vi "Userinterface_BP_MC1.vi"() -> ()   [LabVIEW 2010]
uses:
  <vilib>/addons/Simulation Interface/_sitctls/sit Indicator Info.ctl
  <vilib>/addons/Simulation Interface/_sitctls/sit Indicator Type.ctl
  <vilib>/addons/Simulation Interface/_sitctls/sit Client Meta Info (v3).ctl
  <vilib>/addons/Simulation Interface/_sitctls/sit MDL Line Item Info.ctl
  <vilib>/addons/Simulation Interface/_sitctls/sit MDL Line Type.ctl
  <vilib>/addons/Simulation Interface/_sitctls/sit Details Settings.ctl
  <vilib>/addons/Simulation Interface/_sitctls/sit Execution Host.ctl
  <vilib>/addons/Simulation Interface/_sitctls/SIT Sim State.ctl
  <vilib>/Utility/inputDevices.llb/closeJoystick.vi
  <vilib>/Utility/inputDevices.llb/joystickAcquire.vi
  <vilib>/addons/Simulation Interface/_sitclient.llb/NI_SIT_sitclient.lvlib
  <vilib>/addons/Simulation Interface/_sitctls/NI_SIT_sitctls.lvlib
  <vilib>/ptbypt/NI_PtbyPt.lvlib
panel:
  out "Left Joystick":bool
  out "Right Joystick":bool
  in  "R2":sgl
  in  "L2":sgl
  out "Direction Up":bool
  out "Direction Right":bool
  out "Direction Down":bool
  out "Direction Left":bool
  out "L2 Button":bool
  out "R2 Button":bool
  out "Triangle Button":bool
  out "Circle Button":bool
  out "X Button":bool
  out "Square Button":bool
  out "Joystick Info":T1(array[cluster])
  in  "VSP Speed":dbl(slide) min=-1.0 max=1.0 step=0.05 scale=-1.0..1.0 scale format="%#_2g"
  in  "Power Limiter":dbl(slide) min=0.0 max=1.0 step=0.1 scale=-1.0..1.0
  in  "Left Y":dbl(slide) scale=-35860.0..35860.0
  in  "Left X":dbl(slide) scale=-35860.0..35860.0
  in  "Right X":dbl(slide) scale=-35860.0..35860.0
  in  "Right Y":dbl(slide) scale=-35860.0..35860.0
  in  "SIT_Meta_Info":T2={"Simulation IP"="localhost", "Target IP"="192.168.0.77", "Host Port"=6011, "Model DLL Path"=path "C:/Documents and Settings/mcl/Desktop/CSE Manual Controll/BP_MC1_nidll_rtw/BP_MC1.dll", "Model File Path"=path "C:/Documents and Settings/mcl/Desktop/CSE Manual Controll/BP_MC1_nidll_rtw/BP_MC1.dll", "Model Name"="bp_mc1", "Param Tree Info "=[{"Line Type"=enum."Section Head", "Section Type"="Model", "Name"="bp_mc1", "Value"="", "Owner Index"=-3, "Tree Tag"="", "Child Indices"=[1, 6, 27], "Expanded?"=FALSE, "Destination Block Info"=[]}, {"Line Type"=enum."Section Head", "Section Type"="Subsystem", "Name"="Labview Output", "Value"="", "Owner Index"=0, "Tree Tag"="", "Child Indices"=[2, 4], "Expanded?"=FALSE, "Destination Block Info"=[]}, {"Line Type"=enum."Section Head", "Section Type"="Subsystem", "Name"="LabVIEW_BT_Limit", "Value"="", "Owner Index"=1, "Tree Tag"="", "Child Indices"=[3], "Expanded?"=FALSE, "Destination Block Info"=[]}, {"Line Type"=enum."Parameter", "Section Type"="", "Name"="Value", "Value"="", "Owner Index"=2, "Tree Tag"="", "Child Indices"=[], "Expanded?"=FALSE, "Destination Block Info"=[]}, {"Line Type"=enum."Section Head", "Section Type"="Subsystem", "Name"="LabVIEW_VSPS", "Value"="", "Owner Index"=1, "Tree Tag"="", "Child Indices"=[5], "Expanded?"=FALSE, "Destination Block Info"=[]}, {"Line Type"=enum."Parameter", "Section Type"="", "Name"="Value", "Value"="", "Owner Index"=4, "Tree Tag"="", "Child Indices"=[], "Expanded?"=FALSE, "Destination Block Info"=[]}, {"Line Type"=enum."Section Head", "Section Type"="Subsystem", "Name"="PS3 Controller Output", "Value"="", "Owner Index"=0, "Tree Tag"="", "Child Indices"=[7, 9, 11, 13, 15, 17, 19, 21, 23, 25], "Expanded?"=FALSE, "Destination Block Info"=[]}, {"Line Type"=enum."Section Head", "Section Type"="Subsystem", "Name"="JS_L_X", "Value"="", "Owner Index"=6, "Tree Tag"="", "Child Indices"=[8], "Expanded?"=FALSE, "Destination Block Info"=[]}, {"Line Type"=enum."Parameter", "Section Type"="", "Name"="Value", "Value"="", "Owner Index"=7, "Tree Tag"="", "Child Indices"=[], "Expanded?"=FALSE, "Destination Block Info"=[]}, {"Line Type"=enum."Section Head", "Section Type"="Subsystem", "Name"="JS_L_Y", "Value"="", "Owner Index"=6, "Tree Tag"="", "Child Indices"=[10], "Expanded?"=FALSE, "Destination Block Info"=[]}, {"Line Type"=enum."Parameter", "Section Type"="", "Name"="Value", "Value"="", "Owner Index"=9, "Tree Tag"="", "Child Indices"=[], "Expanded?"=FALSE, "Destination Block Info"=[]}, {"Line Type"=enum."Section Head", "Section Type"="Subsystem", "Name"="JS_R_X", "Value"="", "Owner Index"=6, "Tree Tag"="", "Child Indices"=[12], "Expanded?"=FALSE, "Destination Block Info"=[]}, {"Line Type"=enum."Parameter", "Section Type"="", "Name"="Value", "Value"="", "Owner Index"=11, "Tree Tag"="", "Child Indices"=[], "Expanded?"=FALSE, "Destination Block Info"=[]}, {"Line Type"=enum."Section Head", "Section Type"="Subsystem", "Name"="JS_R_Y", "Value"="", "Owner Index"=6, "Tree Tag"="", "Child Indices"=[14], "Expanded?"=FALSE, "Destination Block Info"=[]}, {"Line Type"=enum."Parameter", "Section Type"="", "Name"="Value", "Value"="", "Owner Index"=13, "Tree Tag"="", "Child Indices"=[], "Expanded?"=FALSE, "Destination Block Info"=[]}, {"Line Type"=enum."Section Head", "Section Type"="Subsystem", "Name"="L2", "Value"="", "Owner Index"=6, "Tree Tag"="", "Child Indices"=[16], "Expanded?"=FALSE, "Destination Block Info"=[]}, {"Line Type"=enum."Parameter", "Section Type"="", "Name"="Value", "Value"="", "Owner Index"=15, "Tree Tag"="", "Child Indices"=[], "Expanded?"=FALSE, "Destination Block Info"=[]}, {"Line Type"=enum."Section Head", "Section Type"="Subsystem", "Name"="R2", "Value"="", "Owner Index"=6, "Tree Tag"="", "Child Indices"=[18], "Expanded?"=FALSE, "Destination Block Info"=[]}, {"Line Type"=enum."Parameter", "Section Type"="", "Name"="Value", "Value"="", "Owner Index"=17, "Tree Tag"="", "Child Indices"=[], "Expanded?"=FALSE, "Destination Block Info"=[]}, {"Line Type"=enum."Section Head", "Section Type"="Subsystem", "Name"="Scaling_JS_L_X", "Value"="", "Owner Index"=6, "Tree Tag"="", "Child Indices"=[20], "Expanded?"=FALSE, "Destination Block Info"=[]}, {"Line Type"=enum."Parameter", "Section Type"="", "Name"="Gain", "Value"="", "Owner Index"=19, "Tree Tag"="", "Child Indices"=[], "Expanded?"=FALSE, "Destination Block Info"=[]}, {"Line Type"=enum."Section Head", "Section Type"="Subsystem", "Name"="Scaling_JS_L_Y", "Value"="", "Owner Index"=6, "Tree Tag"="", "Child Indices"=[22], "Expanded?"=FALSE, "Destination Block Info"=[]}, {"Line Type"=enum."Parameter", "Section Type"="", "Name"="Gain", "Value"="", "Owner Index"=21, "Tree Tag"="", "Child Indices"=[], "Expanded?"=FALSE, "Destination Block Info"=[]}, {"Line Type"=enum."Section Head", "Section Type"="Subsystem", "Name"="Scaling_JS_R_X", "Value"="", "Owner Index"=6, "Tree Tag"="", "Child Indices"=[24], "Expanded?"=FALSE, "Destination Block Info"=[]}, {"Line Type"=enum."Parameter", "Section Type"="", "Name"="Gain", "Value"="", "Owner Index"=23, "Tree Tag"="", "Child Indices"=[], "Expanded?"=FALSE, "Destination Block Info"=[]}, {"Line Type"=enum."Section Head", "Section Type"="Subsystem", "Name"="Scaling_JS_R_Y", "Value"="", "Owner Index"=6, "Tree Tag"="", "Child Indices"=[26], "Expanded?"=FALSE, "Destination Block Info"=[]}, {"Line Type"=enum."Parameter", "Section Type"="", "Name"="Gain", "Value"="", "Owner Index"=25, "Tree Tag"="", "Child Indices"=[], "Expanded?"=FALSE, "Destination Block Info"=[]}, {"Line Type"=enum."Section Head", "Section Type"="Subsystem", "Name"="Thurster Allocation", "Value"="", "Owner Index"=0, "Tree Tag"="", "Child Indices"=[28, 30, 32, 34, 36, 38, 40, 42, 44, 46, 50, 54, 58, 62, 64], "Expanded?"=FALSE, "Destination Block Info"=[]}, {"Line Type"=enum."Section Head", "Section Type"="Subsystem", "Name"="BT_D_Gain1", "Value"="", "Owner Index"=27, "Tree Tag"="", "Child Indices"=[29], "Expanded?"=FALSE, "Destination Block Info"=[]}, {"Line Type"=enum."Parameter", "Section Type"="", "Name"="Gain", "Value"="", "Owner Index"=28, "Tree Tag"="", "Child Indices"=[], "Expanded?"=FALSE, "Destination Block Info"=[]}, {"Line Type"=enum."Section Head", "Section Type"="Subsystem", "Name"="BT_D_Gain2", "Value"="", "Owner Index"=27, "Tree Tag"="", "Child Indices"=[31], "Expanded?"=FALSE, "Destination Block Info"=[]}, {"Line Type"=enum."Parameter", "Section Type"="", "Name"="Gain", "Value"="", "Owner Index"=30, "Tree Tag"="", "Child Indices"=[], "Expanded?"=FALSE, "Destination Block Info"=[]}, {"Line Type"=enum."Section Head", "Section Type"="Subsystem", "Name"="BT_L_Gain1", "Value"="", "Owner Index"=27, "Tree Tag"="", "Child Indices"=[33], "Expanded?"=FALSE, "Destination Block Info"=[]}, {"Line Type"=enum."Parameter", "Section Type"="", "Name"="Gain", "Value"="", "Owner Index"=32, "Tree Tag"="", "Child Indices"=[], "Expanded?"=FALSE, "Destination Block Info"=[]}, {"Line Type"=enum."Section Head", "Section Type"="Subsystem", "Name"="BT_L_Gain2", "Value"="", "Owner Index"=27, "Tree Tag"="", "Child Indices"=[35], "Expanded?"=FALSE, "Destination Block Info"=[]}, {"Line Type"=enum."Parameter", "Section Type"="", "Name"="Gain", "Value"="", "Owner Index"=34, "Tree Tag"="", "Child Indices"=[], "Expanded?"=FALSE, "Destination Block Info"=[]}, {"Line Type"=enum."Section Head", "Section Type"="Subsystem", "Name"="BT_Power_Offset1", "Value"="", "Owner Index"=27, "Tree Tag"="", "Child Indices"=[37], "Expanded?"=FALSE, "Destination Block Info"=[]}, {"Line Type"=enum."Parameter", "Section Type"="", "Name"="Value", "Value"="", "Owner Index"=36, "Tree Tag"="", "Child Indices"=[], "Expanded?"=FALSE, "Destination Block Info"=[]}, {"Line Type"=enum."Section Head", "Section Type"="Subsystem", "Name"="BT_Power_Offset2", "Value"="", "Owner Index"=27, "Tree Tag"="", "Child Indices"=[39], "Expanded?"=FALSE, "Destination Block Info"=[]}, {"Line Type"=enum."Parameter", "Section Type"="", "Name"="Value", "Value"="", "Owner Index"=38, "Tree Tag"="", "Child Indices"=[], "Expanded?"=FALSE, "Destination Block Info"=[]}, {"Line Type"=enum."Section Head", "Section Type"="Subsystem", "Name"="BT_Power_Offset3", "Value"="", "Owner Index"=27, "Tree Tag"="", "Child Indices"=[41], "Expanded?"=FALSE, "Destination Block Info"=[]}, {"Line Type"=enum."Parameter", "Section Type"="", "Name"="Value", "Value"="", "Owner Index"=40, "Tree Tag"="", "Child Indices"=[], "Expanded?"=FALSE, "Destination Block Info"=[]}, {"Line Type"=enum."Section Head", "Section Type"="Subsystem", "Name"="Neg1", "Value"="", "Owner Index"=27, "Tree Tag"="", "Child Indices"=[43], "Expanded?"=FALSE, "Destination Block Info"=[]}, {"Line Type"=enum."Parameter", "Section Type"="", "Name"="Gain", "Value"="", "Owner Index"=42, "Tree Tag"="", "Child Indices"=[], "Expanded?"=FALSE, "Destination Block Info"=[]}, {"Line Type"=enum."Section Head", "Section Type"="Subsystem", "Name"="Neg2", "Value"="", "Owner Index"=27, "Tree Tag"="", "Child Indices"=[45], "Expanded?"=FALSE, "Destination Block Info"=[]}, {"Line Type"=enum."Parameter", "Section Type"="", "Name"="Gain", "Value"="", "Owner Index"=44, "Tree Tag"="", "Child Indices"=[], "Expanded?"=FALSE, "Destination Block Info"=[]}, {"Line Type"=enum."Section Head", "Section Type"="Subsystem", "Name"="Servo1", "Value"="", "Owner Index"=27, "Tree Tag"="", "Child Indices"=[47, 48, 49], "Expanded?"=FALSE, "Destination Block Info"=[]}, {"Line Type"=enum."Parameter", "Section Type"="", "Name"="ColumnIndex", "Value"="", "Owner Index"=46, "Tree Tag"="", "Child Indices"=[], "Expanded?"=FALSE, "Destination Block Info"=[]}, {"Line Type"=enum."Parameter", "Section Type"="", "Name"="RowIndex", "Value"="", "Owner Index"=46, "Tree Tag"="", "Child Indices"=[], "Expanded?"=FALSE, "Destination Block Info"=[]}, {"Line Type"=enum."Parameter", "Section Type"="", "Name"="Table", "Value"="", "Owner Index"=46, "Tree Tag"="", "Child Indices"=[], "Expanded?"=FALSE, "Destination Block Info"=[]}, {"Line Type"=enum."Section Head", "Section Type"="Subsystem", "Name"="Servo2", "Value"="", "Owner Index"=27, "Tree Tag"="", "Child Indices"=[51, 52, 53], "Expanded?"=FALSE, "Destination Block Info"=[]}, {"Line Type"=enum."Parameter", "Section Type"="", "Name"="ColumnIndex", "Value"="", "Owner Index"=50, "Tree Tag"="", "Child Indices"=[], "Expanded?"=FALSE, "Destination Block Info"=[]}, {"Line Type"=enum."Parameter", "Section Type"="", "Name"="RowIndex", "Value"="", "Owner Index"=50, "Tree Tag"="", "Child Indices"=[], "Expanded?"=FALSE, "Destination Block Info"=[]}, {"Line Type"=enum."Parameter", "Section Type"="", "Name"="Table", "Value"="", "Owner Index"=50, "Tree Tag"="", "Child Indices"=[], "Expanded?"=FALSE, "Destination Block Info"=[]}, {"Line Type"=enum."Section Head", "Section Type"="Subsystem", "Name"="Servo3", "Value"="", "Owner Index"=27, "Tree Tag"="", "Child Indices"=[55, 56, 57], "Expanded?"=FALSE, "Destination Block Info"=[]}, {"Line Type"=enum."Parameter", "Section Type"="", "Name"="ColumnIndex", "Value"="", "Owner Index"=54, "Tree Tag"="", "Child Indices"=[], "Expanded?"=FALSE, "Destination Block Info"=[]}, {"Line Type"=enum."Parameter", "Section Type"="", "Name"="RowIndex", "Value"="", "Owner Index"=54, "Tree Tag"="", "Child Indices"=[], "Expanded?"=FALSE, "Destination Block Info"=[]}, {"Line Type"=enum."Parameter", "Section Type"="", "Name"="Table", "Value"="", "Owner Index"=54, "Tree Tag"="", "Child Indices"=[], "Expanded?"=FALSE, "Destination Block Info"=[]}, {"Line Type"=enum."Section Head", "Section Type"="Subsystem", "Name"="Servo4", "Value"="", "Owner Index"=27, "Tree Tag"="", "Child Indices"=[59, 60, 61], "Expanded?"=FALSE, "Destination Block Info"=[]}, {"Line Type"=enum."Parameter", "Section Type"="", "Name"="ColumnIndex", "Value"="", "Owner Index"=58, "Tree Tag"="", "Child Indices"=[], "Expanded?"=FALSE, "Destination Block Info"=[]}, {"Line Type"=enum."Parameter", "Section Type"="", "Name"="RowIndex", "Value"="", "Owner Index"=58, "Tree Tag"="", "Child Indices"=[], "Expanded?"=FALSE, "Destination Block Info"=[]}, {"Line Type"=enum."Parameter", "Section Type"="", "Name"="Table", "Value"="", "Owner Index"=58, "Tree Tag"="", "Child Indices"=[], "Expanded?"=FALSE, "Destination Block Info"=[]}, {"Line Type"=enum."Section Head", "Section Type"="Subsystem", "Name"="VPS_Power_Offset", "Value"="", "Owner Index"=27, "Tree Tag"="", "Child Indices"=[63], "Expanded?"=FALSE, "Destination Block Info"=[]}, {"Line Type"=enum."Parameter", "Section Type"="", "Name"="Value", "Value"="", "Owner Index"=62, "Tree Tag"="", "Child Indices"=[], "Expanded?"=FALSE, "Destination Block Info"=[]}, {"Line Type"=enum."Section Head", "Section Type"="Subsystem", "Name"="VPS_Speed_Gain", "Value"="", "Owner Index"=27, "Tree Tag"="", "Child Indices"=[65], "Expanded?"=FALSE, "Destination Block Info"=[]}, {"Line Type"=enum."Parameter", "Section Type"="", "Name"="Gain", "Value"="", "Owner Index"=64, "Tree Tag"="", "Child Indices"=[], "Expanded?"=FALSE, "Destination Block Info"=[]}], "Signal Tree Info"=[{"Line Type"=enum."Section Head", "Section Type"="Model", "Name"="bp_mc1", "Value"="", "Owner Index"=-3, "Tree Tag"="", "Child Indices"=[1, 4, 13], "Expanded?"=FALSE, "Destination Block Info"=[]}, {"Line Type"=enum."Section Head", "Section Type"="Subsystem", "Name"="Manual Thrust controll", "Value"="", "Owner Index"=0, "Tree Tag"="", "Child Indices"=[2], "Expanded?"=FALSE, "Destination Block Info"=[]}, {"Line Type"=enum."Section Head", "Section Type"="Subsystem", "Name"="Add", "Value"="", "Owner Index"=1, "Tree Tag"="", "Child Indices"=[3], "Expanded?"=FALSE, "Destination Block Info"=[]}, {"Line Type"=enum."Parameter", "Section Type"="", "Name"="Port 1", "Value"="Bow Thruster direction", "Owner Index"=2, "Tree Tag"="", "Child Indices"=[], "Expanded?"=FALSE, "Destination Block Info"=[]}, {"Line Type"=enum."Section Head", "Section Type"="Subsystem", "Name"="PS3 Controller Output", "Value"="", "Owner Index"=0, "Tree Tag"="", "Child Indices"=[5, 7, 9, 11], "Expanded?"=FALSE, "Destination Block Info"=[]}, {"Line Type"=enum."Section Head", "Section Type"="Subsystem", "Name"="Scaling_JS_L_X", "Value"="", "Owner Index"=4, "Tree Tag"="", "Child Indices"=[6], "Expanded?"=FALSE, "Destination Block Info"=[]}, {"Line Type"=enum."Parameter", "Section Type"="", "Name"="Port 1", "Value"="[-1,1]", "Owner Index"=5, "Tree Tag"="", "Child Indices"=[], "Expanded?"=FALSE, "Destination Block Info"=[]}, {"Line Type"=enum."Section Head", "Section Type"="Subsystem", "Name"="Scaling_JS_L_Y", "Value"="", "Owner Index"=4, "Tree Tag"="", "Child Indices"=[8], "Expanded?"=FALSE, "Destination Block Info"=[]}, {"Line Type"=enum."Parameter", "Section Type"="", "Name"="Port 1", "Value"="[-1,1]", "Owner Index"=7, "Tree Tag"="", "Child Indices"=[], "Expanded?"=FALSE, "Destination Block Info"=[]}, {"Line Type"=enum."Section Head", "Section Type"="Subsystem", "Name"="Scaling_JS_R_X", "Value"="", "Owner Index"=4, "Tree Tag"="", "Child Indices"=[10], "Expanded?"=FALSE, "Destination Block Info"=[]}, {"Line Type"=enum."Parameter", "Section Type"="", "Name"="Port 1", "Value"="[-1,1]", "Owner Index"=9, "Tree Tag"="", "Child Indices"=[], "Expanded?"=FALSE, "Destination Block Info"=[]}, {"Line Type"=enum."Section Head", "Section Type"="Subsystem", "Name"="Scaling_JS_R_Y", "Value"="", "Owner Index"=4, "Tree Tag"="", "Child Indices"=[12], "Expanded?"=FALSE, "Destination Block Info"=[]}, {"Line Type"=enum."Parameter", "Section Type"="", "Name"="Port 1", "Value"="[-1,1]", "Owner Index"=11, "Tree Tag"="", "Child Indices"=[], "Expanded?"=FALSE, "Destination Block Info"=[]}, {"Line Type"=enum."Section Head", "Section Type"="Subsystem", "Name"="Thurster Allocation", "Value"="", "Owner Index"=0, "Tree Tag"="", "Child Indices"=[14, 16, 18, 20, 22, 24, 26, 28, 30, 32, 34, 36, 45, 47, 49, 51, 53, 55, 57, 59, 61], "Expanded?"=FALSE, "Destination Block Info"=[]}, {"Line Type"=enum."Section Head", "Section Type"="Subsystem", "Name"="Add", "Value"="", "Owner Index"=13, "Tree Tag"="", "Child Indices"=[15], "Expanded?"=FALSE, "Destination Block Info"=[]}, {"Line Type"=enum."Parameter", "Section Type"="", "Name"="Port 1", "Value"="", "Owner Index"=14, "Tree Tag"="", "Child Indices"=[], "Expanded?"=FALSE, "Destination Block Info"=[]}, {"Line Type"=enum."Section Head", "Section Type"="Subsystem", "Name"="BT_D_Gain1", "Value"="", "Owner Index"=13, "Tree Tag"="", "Child Indices"=[17], "Expanded?"=FALSE, "Destination Block Info"=[]}, {"Line Type"=enum."Parameter", "Section Type"="", "Name"="Port 1", "Value"="", "Owner Index"=16, "Tree Tag"="", "Child Indices"=[], "Expanded?"=FALSE, "Destination Block Info"=[]}, {"Line Type"=enum."Section Head", "Section Type"="Subsystem", "Name"="BT_D_Gain2", "Value"="", "Owner Index"=13, "Tree Tag"="", "Child Indices"=[19], "Expanded?"=FALSE, "Destination Block Info"=[]}, {"Line Type"=enum."Parameter", "Section Type"="", "Name"="Port 1", "Value"="", "Owner Index"=18, "Tree Tag"="", "Child Indices"=[], "Expanded?"=FALSE, "Destination Block Info"=[]}, {"Line Type"=enum."Section Head", "Section Type"="Subsystem", "Name"="BT_L_Gain1", "Value"="", "Owner Index"=13, "Tree Tag"="", "Child Indices"=[21], "Expanded?"=FALSE, "Destination Block Info"=[]}, {"Line Type"=enum."Parameter", "Section Type"="", "Name"="Port 1", "Value"="", "Owner Index"=20, "Tree Tag"="", "Child Indices"=[], "Expanded?"=FALSE, "Destination Block Info"=[]}, {"Line Type"=enum."Section Head", "Section Type"="Subsystem", "Name"="BT_L_Gain2", "Value"="", "Owner Index"=13, "Tree Tag"="", "Child Indices"=[23], "Expanded?"=FALSE, "Destination Block Info"=[]}, {"Line Type"=enum."Parameter", "Section Type"="", "Name"="Port 1", "Value"="", "Owner Index"=22, "Tree Tag"="", "Child Indices"=[], "Expanded?"=FALSE, "Destination Block Info"=[]}, {"Line Type"=enum."Section Head", "Section Type"="Subsystem", "Name"="Neg1", "Value"="", "Owner Index"=13, "Tree Tag"="", "Child Indices"=[25], "Expanded?"=FALSE, "Destination Block Info"=[]}, {"Line Type"=enum."Parameter", "Section Type"="", "Name"="Port 1", "Value"="Port VPS_X", "Owner Index"=24, "Tree Tag"="", "Child Indices"=[], "Expanded?"=FALSE, "Destination Block Info"=[]}, {"Line Type"=enum."Section Head", "Section Type"="Subsystem", "Name"="Neg2", "Value"="", "Owner Index"=13, "Tree Tag"="", "Child Indices"=[27], "Expanded?"=FALSE, "Destination Block Info"=[]}, {"Line Type"=enum."Parameter", "Section Type"="", "Name"="Port 1", "Value"="Port VSP_Y", "Owner Index"=26, "Tree Tag"="", "Child Indices"=[], "Expanded?"=FALSE, "Destination Block Info"=[]}, {"Line Type"=enum."Section Head", "Section Type"="Subsystem", "Name"="Product1", "Value"="", "Owner Index"=13, "Tree Tag"="", "Child Indices"=[29], "Expanded?"=FALSE, "Destination Block Info"=[]}, {"Line Type"=enum."Parameter", "Section Type"="", "Name"="Port 1", "Value"="Port VPS_X", "Owner Index"=28, "Tree Tag"="", "Child Indices"=[], "Expanded?"=FALSE, "Destination Block Info"=[]}, {"Line Type"=enum."Section Head", "Section Type"="Subsystem", "Name"="Product2", "Value"="", "Owner Index"=13, "Tree Tag"="", "Child Indices"=[31], "Expanded?"=FALSE, "Destination Block Info"=[]}, {"Line Type"=enum."Parameter", "Section Type"="", "Name"="Port 1", "Value"="Port VSP_Y", "Owner Index"=30, "Tree Tag"="", "Child Indices"=[], "Expanded?"=FALSE, "Destination Block Info"=[]}, {"Line Type"=enum."Section Head", "Section Type"="Subsystem", "Name"="Product3", "Value"="", "Owner Index"=13, "Tree Tag"="", "Child Indices"=[33], "Expanded?"=FALSE, "Destination Block Info"=[]}, {"Line Type"=enum."Parameter", "Section Type"="", "Name"="Port 1", "Value"="Starboard VSP_X", "Owner Index"=32, "Tree Tag"="", "Child Indices"=[], "Expanded?"=FALSE, "Destination Block Info"=[]}, {"Line Type"=enum."Section Head", "Section Type"="Subsystem", "Name"="Product4", "Value"="", "Owner Index"=13, "Tree Tag"="", "Child Indices"=[35], "Expanded?"=FALSE, "Destination Block Info"=[]}, {"Line Type"=enum."Parameter", "Section Type"="", "Name"="Port 1", "Value"="Starboard VSP_Y", "Owner Index"=34, "Tree Tag"="", "Child Indices"=[], "Expanded?"=FALSE, "Destination Block Info"=[]}, {"Line Type"=enum."Section Head", "Section Type"="Subsystem", "Name"="Saturation Dynamic", "Value"="", "Owner Index"=13, "Tree Tag"="", "Child Indices"=[37, 39, 41, 43], "Expanded?"=FALSE, "Destination Block Info"=[]}, {"Line Type"=enum."Section Head", "Section Type"="Subsystem", "Name"="LowerRelop1", "Value"="", "Owner Index"=36, "Tree Tag"="", "Child Indices"=[38], "Expanded?"=FALSE, "Destination Block Info"=[]}, {"Line Type"=enum."Parameter", "Section Type"="", "Name"="Port 1", "Value"="", "Owner Index"=37, "Tree Tag"="", "Child Indices"=[], "Expanded?"=FALSE, "Destination Block Info"=[]}, {"Line Type"=enum."Section Head", "Section Type"="Subsystem", "Name"="Switch", "Value"="", "Owner Index"=36, "Tree Tag"="", "Child Indices"=[40], "Expanded?"=FALSE, "Destination Block Info"=[]}, {"Line Type"=enum."Parameter", "Section Type"="", "Name"="Port 1", "Value"="", "Owner Index"=39, "Tree Tag"="", "Child Indices"=[], "Expanded?"=FALSE, "Destination Block Info"=[]}, {"Line Type"=enum."Section Head", "Section Type"="Subsystem", "Name"="Switch2", "Value"="", "Owner Index"=36, "Tree Tag"="", "Child Indices"=[42], "Expanded?"=FALSE, "Destination Block Info"=[]}, {"Line Type"=enum."Parameter", "Section Type"="", "Name"="Port 1", "Value"="", "Owner Index"=41, "Tree Tag"="", "Child Indices"=[], "Expanded?"=FALSE, "Destination Block Info"=[]}, {"Line Type"=enum."Section Head", "Section Type"="Subsystem", "Name"="UpperRelop", "Value"="", "Owner Index"=36, "Tree Tag"="", "Child Indices"=[44], "Expanded?"=FALSE, "Destination Block Info"=[]}, {"Line Type"=enum."Parameter", "Section Type"="", "Name"="Port 1", "Value"="", "Owner Index"=43, "Tree Tag"="", "Child Indices"=[], "Expanded?"=FALSE, "Destination Block Info"=[]}, {"Line Type"=enum."Section Head", "Section Type"="Subsystem", "Name"="Servo1", "Value"="", "Owner Index"=13, "Tree Tag"="", "Child Indices"=[46], "Expanded?"=FALSE, "Destination Block Info"=[]}, {"Line Type"=enum."Parameter", "Section Type"="", "Name"="Port 1", "Value"="", "Owner Index"=45, "Tree Tag"="", "Child Indices"=[], "Expanded?"=FALSE, "Destination Block Info"=[]}, {"Line Type"=enum."Section Head", "Section Type"="Subsystem", "Name"="Servo2", "Value"="", "Owner Index"=13, "Tree Tag"="", "Child Indices"=[48], "Expanded?"=FALSE, "Destination Block Info"=[]}, {"Line Type"=enum."Parameter", "Section Type"="", "Name"="Port 1", "Value"="", "Owner Index"=47, "Tree Tag"="", "Child Indices"=[], "Expanded?"=FALSE, "Destination Block Info"=[]}, {"Line Type"=enum."Section Head", "Section Type"="Subsystem", "Name"="Servo3", "Value"="", "Owner Index"=13, "Tree Tag"="", "Child Indices"=[50], "Expanded?"=FALSE, "Destination Block Info"=[]}, {"Line Type"=enum."Parameter", "Section Type"="", "Name"="Port 1", "Value"="", "Owner Index"=49, "Tree Tag"="", "Child Indices"=[], "Expanded?"=FALSE, "Destination Block Info"=[]}, {"Line Type"=enum."Section Head", "Section Type"="Subsystem", "Name"="Servo4", "Value"="", "Owner Index"=13, "Tree Tag"="", "Child Indices"=[52], "Expanded?"=FALSE, "Destination Block Info"=[]}, {"Line Type"=enum."Parameter", "Section Type"="", "Name"="Port 1", "Value"="", "Owner Index"=51, "Tree Tag"="", "Child Indices"=[], "Expanded?"=FALSE, "Destination Block Info"=[]}, {"Line Type"=enum."Section Head", "Section Type"="Subsystem", "Name"="Sign", "Value"="", "Owner Index"=13, "Tree Tag"="", "Child Indices"=[54], "Expanded?"=FALSE, "Destination Block Info"=[]}, {"Line Type"=enum."Parameter", "Section Type"="", "Name"="Port 1", "Value"="", "Owner Index"=53, "Tree Tag"="", "Child Indices"=[], "Expanded?"=FALSE, "Destination Block Info"=[]}, {"Line Type"=enum."Section Head", "Section Type"="Subsystem", "Name"="Sum", "Value"="", "Owner Index"=13, "Tree Tag"="", "Child Indices"=[56], "Expanded?"=FALSE, "Destination Block Info"=[]}, {"Line Type"=enum."Parameter", "Section Type"="", "Name"="Port 1", "Value"="", "Owner Index"=55, "Tree Tag"="", "Child Indices"=[], "Expanded?"=FALSE, "Destination Block Info"=[]}, {"Line Type"=enum."Section Head", "Section Type"="Subsystem", "Name"="Sum1", "Value"="", "Owner Index"=13, "Tree Tag"="", "Child Indices"=[58], "Expanded?"=FALSE, "Destination Block Info"=[]}, {"Line Type"=enum."Parameter", "Section Type"="", "Name"="Port 1", "Value"="", "Owner Index"=57, "Tree Tag"="", "Child Indices"=[], "Expanded?"=FALSE, "Destination Block Info"=[]}, {"Line Type"=enum."Section Head", "Section Type"="Subsystem", "Name"="Sum2", "Value"="", "Owner Index"=13, "Tree Tag"="", "Child Indices"=[60], "Expanded?"=FALSE, "Destination Block Info"=[]}, {"Line Type"=enum."Parameter", "Section Type"="", "Name"="Port 1", "Value"="", "Owner Index"=59, "Tree Tag"="", "Child Indices"=[], "Expanded?"=FALSE, "Destination Block Info"=[]}, {"Line Type"=enum."Section Head", "Section Type"="Subsystem", "Name"="VPS_Speed_Gain", "Value"="", "Owner Index"=13, "Tree Tag"="", "Child Indices"=[62], "Expanded?"=FALSE, "Destination Block Info"=[]}, {"Line Type"=enum."Parameter", "Section Type"="", "Name"="Port 1", "Value"="", "Owner Index"=61, "Tree Tag"="", "Child Indices"=[], "Expanded?"=FALSE, "Destination Block Info"=[]}], "Details Settings"={"Halt on Task Overrun?"=FALSE, "Halt on Lost Data?"=FALSE, "Signal Decimation"=1, "Autoscale"=FALSE}, "Client Name"="Userinterface_BP_MC1.vi", "Stored Model Checksum"="db0cad4409aaf4382302511f567ab5c4", "Buffer Sizes"={"number of signals"=50, "circular buffer size"=1000, "num data points"=100}, "Execution Host"=enum."RT Target", "Project Dir"=path "C:/Documents and Settings/mcl/Desktop/CSE Manual Controll", "Last MDL"=path "C:/Documents and Settings/namdinh.IIMT-LAB-TWA2/Desktop/Manual Controll/BP_MC1.mdl"}
  in  "SIT_Indicator_Indices":T7[](array[typedef])
  in  "SIT_RVE":bool
  in  "SIT_Remap":bool
  in  "SIT_Details":bool
  in  "SIT_Stop":bool
  in  "SIT_Pause":bool
  in  "SIT_Run":bool
  in  "SIT_stopVI":bool
  out "SIT_Status":string
  # "Model Controls"
  # "VSP Speed"
  # "Starboard full ClockWise\nPort full CounterClockWise"
  # "Increase BT power limit"
  # "Increase VSP speed"
  # "Starboard full CounterClockWise\nPort full ClockWise"
  # "Decrease BT power limit"
  # "Decrease VSP speed"
  # "Bow Thruster Power Limit"
  # "Max Power"
  # "Max Power"
  # "No Power"
  # "PS3 Joysticks"
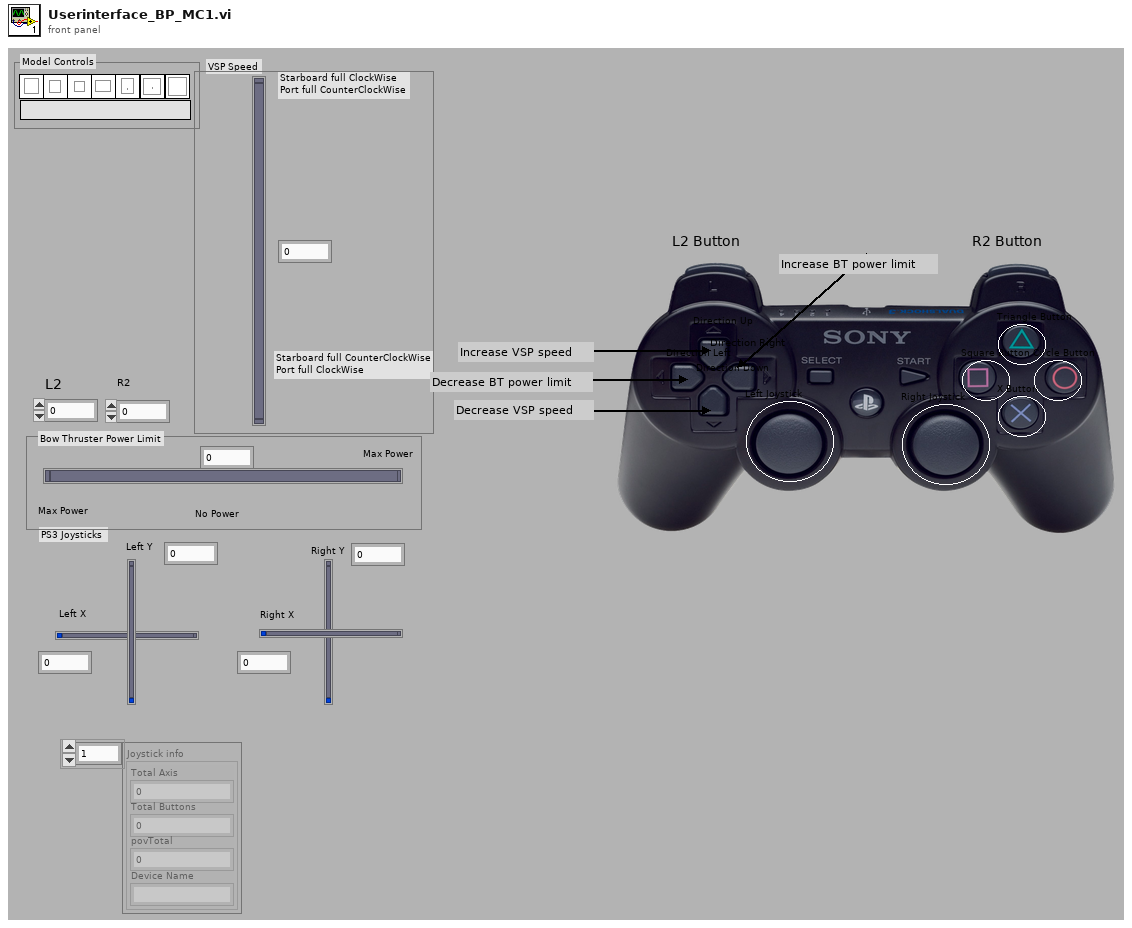
[diagram p1: front panel]
types:
  T1 = cluster{"Total Axis":u32, "Total Buttons":u32, "povTotal":u32, "Device Name":string}[]
  T2 = typedef "NI_SIT_sitctls.lvlib/sit Client Meta Info (v3).ctl" = cluster{"Simulation IP":string, "Target IP":string, "Host Port":u16, "Model DLL Path":path, "Model File Path":path, "Model Name":string, "Param Tree Info ":T3[], "Signal Tree Info":T3[], "Details Settings":T5, "Client Name":string, "Stored Model Checksum":string, "Buffer Sizes":cluster{"number of signals":u32, "circular buffer size":u32, "num data points":u32}, "Execution Host":T6, "Project Dir":path, "Last MDL":path}
  T3 = typedef "NI_SIT_sitctls.lvlib/sit MDL Line Item Info.ctl" = cluster{"Line Type":T4, "Section Type":string, "Name":string, "Value":string, "Owner Index":i32, "Tree Tag":string, "Child Indices":i32[], "Expanded?":bool, "Destination Block Info":string[]}
  T4 = typedef "NI_SIT_sitctls.lvlib/sit MDL Line Type.ctl" = enum16{"Section Head", "Parameter", "Section End", "Comment"}
  T5 = typedef "NI_SIT_sitctls.lvlib/sit Details Settings.ctl" = cluster{"Halt on Task Overrun?":bool, "Halt on Lost Data?":bool, "Signal Decimation":i32, "Autoscale":bool}
  T6 = typedef "NI_SIT_sitctls.lvlib/sit Execution Host.ctl" = enum32{"Simulation Environment", "RT Target", "Local Driver"}
  T7 = typedef "NI_SIT_sitctls.lvlib/sit Indicator Info.ctl" = cluster{"Indicator Index":i32, "Number of Signals":i32, "Indicator Type":T8}
  T8 = typedef "NI_SIT_sitctls.lvlib/sit Indicator Type.ctl" = enum32{"xxx1", "xxx2", "xxx3", "Generic   ", "Decoration", "Text", "xControl", "ColorBox", "Boolean", "RefNum", "Variant", "Path", "ListBox", "Table", "Array", "Picture", "ActiveXContainer", "Numeric", "Digital", "NamedNumeric", "ColorRamp", "Slide", "GraphOrChart", "WaveformChart", "WaveformGraph", "IntensityChart", "xxx4", "xxx5", "xxx6", "xxx7", "Cluster", "Panel", "Knob", "NumWithScale", "Ring", "Enum", "GObject", "Plot", "Cursor", "NumericText", "Scale", "ColorScale", "GraphScale", "ColorGraphScale", "TypedRefNum", "OldKnobScale", "MCListbox", "WaveformData", "BVTag", "DAQName", "VISAName", "IVIName", "SlideScale"}
  T9 = cluster{"axes total":u32, "buttons total":u32, "pov total":u32, "device name":string}[]
  T10 = typedef "NI_SIT_sitctls.lvlib/sit TCP Conn and Queue.ctl" = cluster{"TCP Connection":refnum<k5>, "Data Queue":refnum<queue>, "Execution Host":T6}
  T11 = typedef "NI_SIT_sitctls.lvlib/sit Client Op Refs.ctl" = cluster{"Conn and Queue":T10, "RunPauseStop Refs":refnum<vi>[], "Control Refs":refnum<vi>[], "Indicator Refs":refnum<vi>[], "Param Info":T12[], "State Queue":refnum<queue>, "Don't Modify Scales?":bool, "Param Info Needs Init?":bool}
  T12 = typedef "NI_SIT_sitctls.lvlib/SIT param info.ctl" = cluster{"paramidx":i32, "ID":string, "paramname":string, "dattype":i32, "Dimensions":i32[], "value":dbl[]}
  T13 = typedef "NI_SIT_sitctls.lvlib/SIT Sim State.ctl" = enum8{"Default", "Idle", "Running", "Paused", "Stopped", "Error"}
  T14 = cluster{"X axis":i32, "Y axis":i32, "Z axis":i32, "X axis rotation":i32, "Y axis rotation":i32, "Z axis rotation":i32, "U axis":i32, "V axis":i32}
  T15 = cluster{"button 1":bool, "button 2":bool, "button 3":bool, "button 4":bool, "button 5":bool, "button 6":bool, "button 7":bool, "button 8":bool, "button 9":bool, "button 10":bool, "button 11":bool, "button 12":bool, "button 13":bool, "button 14":bool, "button 15":bool, "button 16":bool, "button 17":bool, "button 18":bool, "button 19":bool, "button 20":bool, "button 21":bool, "button 22":bool, "button 23":bool, "button 24":bool, "button 25":bool, "button 26":bool, "button 27":bool, "button 28":bool, "button 29":bool, "button 30":bool, "button 31":bool, "button 32":bool}
  T16 = cluster{"pov 1":i32, "pov 2":i32, "pov 3":i32, "pov 4":i32}
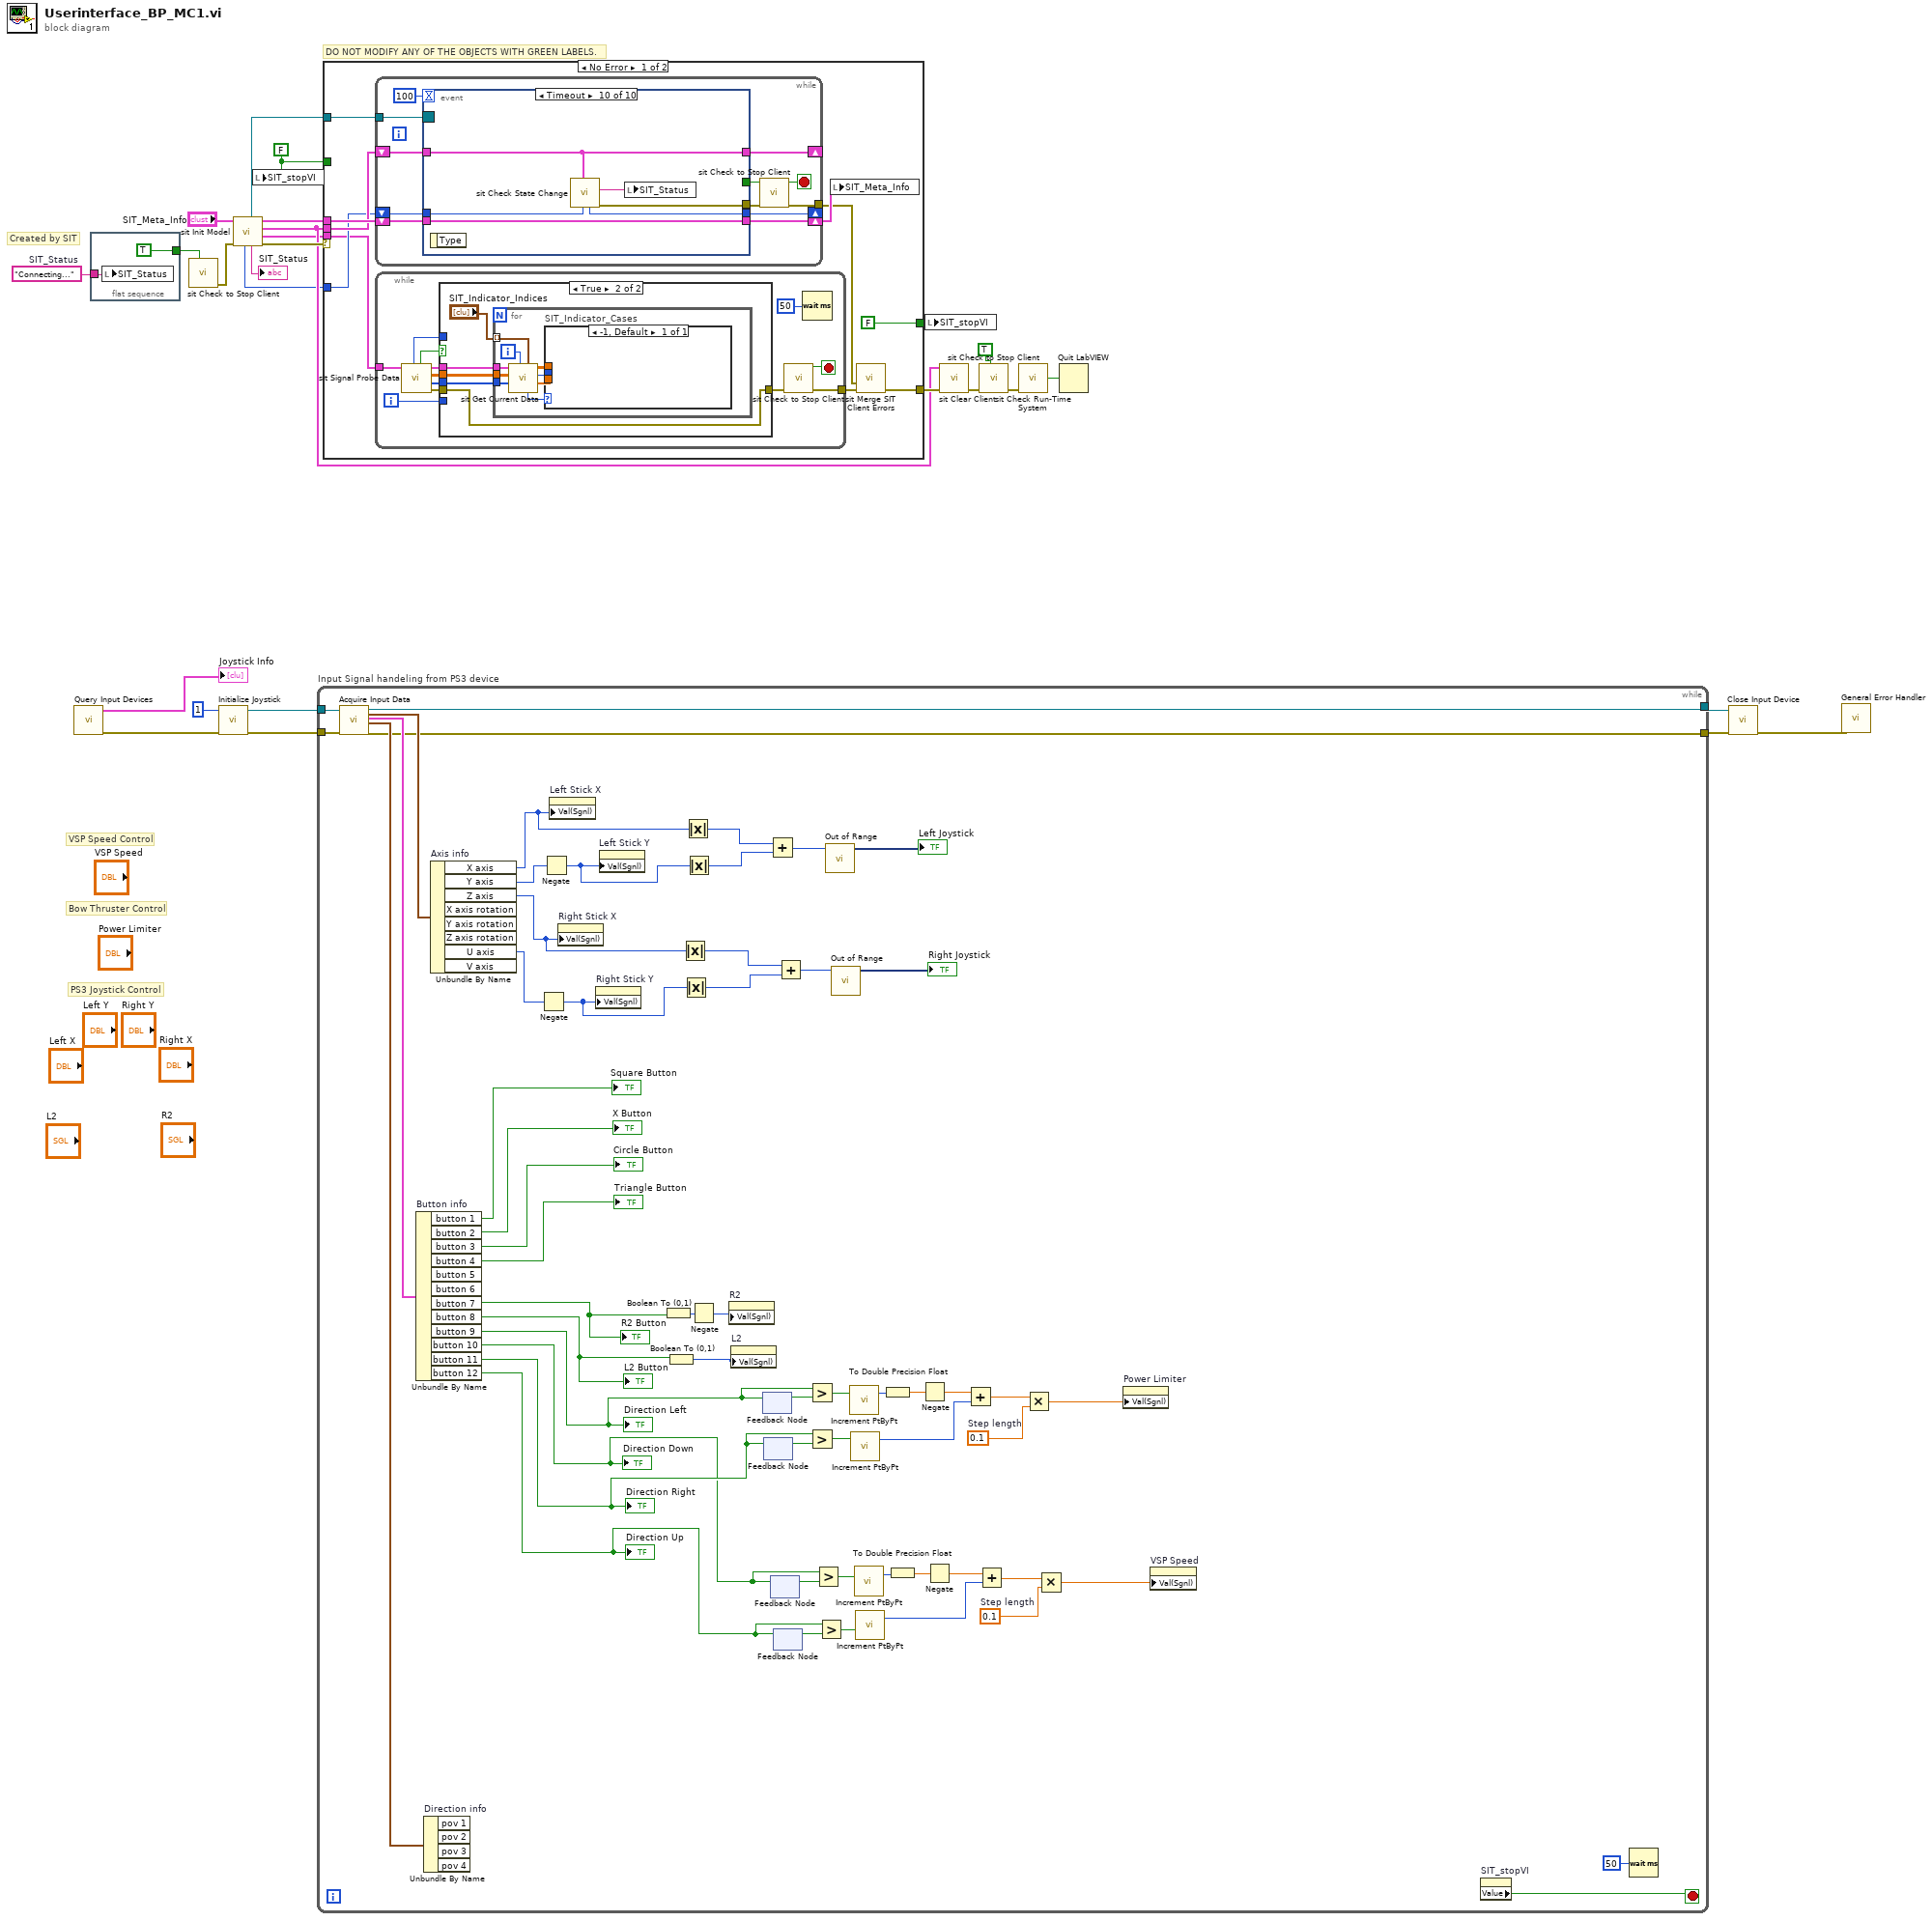
[diagram p0: block diagram]
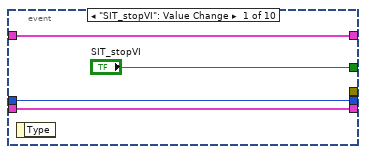
[diagram p2: hidden frame]
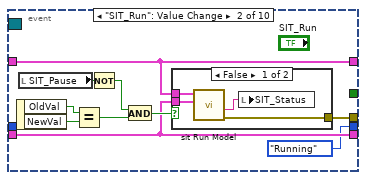
[diagram p3: hidden frame]
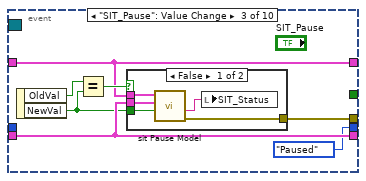
[diagram p5: hidden frame]
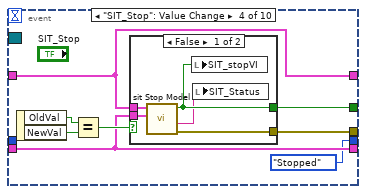
[diagram p7: hidden frame]
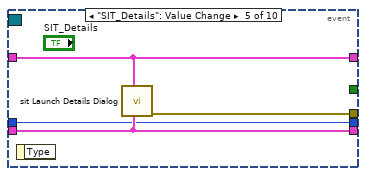
[diagram p9: hidden frame]
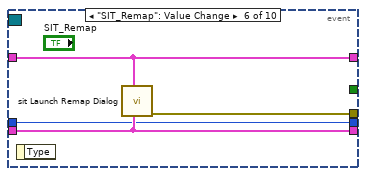
[diagram p10: hidden frame]
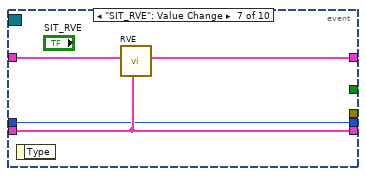
[diagram p11: hidden frame]
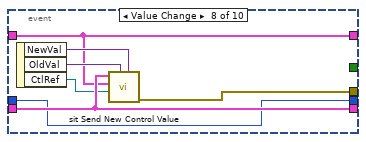
[diagram p12: hidden frame]
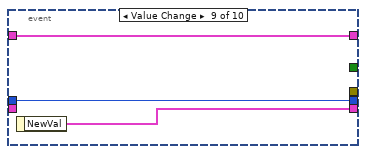
[diagram p13: hidden frame]
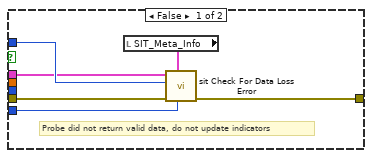
[diagram p14: hidden frame]
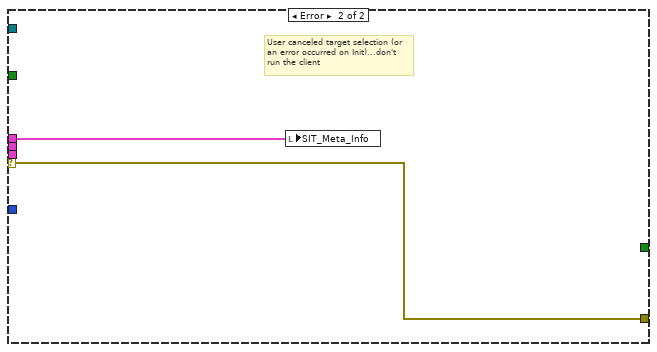
[diagram p15: hidden frame]
diagram:
  w11 = "Connecting..."  # SIT_Status
  w16 = FALSE
  # "VSP Speed Control"
  # "Bow Thruster Control"
  # "Created by SIT"
  # "PS3 Joystick Control"
  # "DO NOT MODIFY ANY OF THE OBJECTS WITH GREEN LABELS."
  n1 = call <vilib>:"Query Input Devices.vi"() -> ("error out"=w5:errorcluster, "joystick info"=→"Joystick Info":T9)  [unwired: 8 in, 2 out]
  n2 = flat-sequence {
    tunnel: [TRUE ("Clear Item?")] -> w20
    tunnel: w11 -> [w27]
    frame #0 {
      n3 = local write "SIT_Status"(w27) -> ()
    }
  }
  n4 = call <vilib>:"sit Check to Stop Client.vi"("Reset Stop?"=w20) -> ("error out"=w22:errorcluster)  [unwired: 2 in, 8 out]
  n5 = call <vilib>:"Initialize Joystick.vi"("error in (no error)"=w5, "device index"=1) -> ("error out"=w7:errorcluster, "device ID"=w8:refnum<k1>)  [unwired: 8 in]
  n6 = call <vilib>:"sit Init Model.vi"("error in (no error)"=w22, "SIT_Meta_Info in"="SIT_Meta_Info") -> ("error out"=w26:errorcluster, "Conn and Queue"=w13:T10, "SIT Client Op Refs"=w17:T11, "SIT_Meta_Info out"=w24:T2, "Initial State"=→"SIT_Status":string, "Event Registration Refnum"=w25:refnum<event-registration>, "State"=w14:T13)  [unwired: 2 in, 1 out]
  n7 = local write "SIT_stopVI"(w16) -> ()
  n8 = while "Input Signal handeling from PS3 device" {
    tunnel: w8 -> [w86]
    tunnel: w7 -> [w85]
    tunnel: [w50] -> w3
    tunnel: [w51] -> w2
    stop <- w36 stop-if-true
    w52 = 0.1  # Step length
    w64 = 0.1  # Step length
    n9 = call-poly <vilib>:"Acquire Input Data.vi"("device ID"=w86, "error in (no error)"=w85) -> ("device ID"=w50:refnum<k1>, "axis info"=w82:T14, "button info"=w84:T15, "direction info"=w83:T16, "error out"=w51:errorcluster)  [unwired: 13 in]
    n10 = Unbundle By Name "Button info"(w84) -> ("button 1"=→"Square Button":bool, "button 2"=→"X Button":bool, "button 3"=→"Circle Button":bool, "button 4"=→"Triangle Button":bool, "button 7"=w34:bool, "button 8"=w35:bool, "button 9"=w68:bool, "button 10"=w56:bool, "button 11"=w67:bool, "button 12"=w55:bool)  [unwired: 2 out]
    "R2 Button" <- w34
    "L2 Button" <- w35
    "Direction Left" <- w68
    "Direction Down" <- w56
    "Direction Right" <- w67
    "Direction Up" <- w55
    n11 = Unbundle By Name "Direction info"(w83) -> ()  [unwired: 4 out]
    n12 = Unbundle By Name "Axis info"(w82) -> ("X axis"=w37:i32, "Y axis"=w81:i32, "Z axis"=w46:i32, "U axis"=w80:i32)  [unwired: 4 out]
    n13 = Negate(x=w80) -> (-x=w45:i32)
    n14 = Negate(x=w81) -> (-x=w38:i32)
    n15 = property on="Left Stick X" class="Slide (strict)"("Val(Sgnl)"=w37) -> ()  [unwired: 2 in, 2 out]
    n16 = property on="Right Stick X" class="Slide (strict)"("Val(Sgnl)"=w46) -> ()  [unwired: 2 in, 2 out]
    n17 = property on="Right Stick Y" class="Slide (strict)"("Val(Sgnl)"=w45) -> ()  [unwired: 2 in, 2 out]
    n18 = property on="Left Stick Y" class="Slide (strict)"("Val(Sgnl)"=w38) -> ()  [unwired: 2 in, 2 out]
    n19 = Boolean To (0,1)(Boolean=w34) -> (0, 1=w33:i16)
    n20 = Boolean To (0,1)(Boolean=w35) -> (0, 1=w30:i16)
    n21 = Absolute Value(x=w46) -> (abs(x)=w43:i32)
    n22 = Absolute Value(x=w45) -> (abs(x)=w44:i32)
    n23 = Absolute Value(x=w37) -> (abs(x)=w40:i32)
    n24 = Absolute Value(x=w38) -> (abs(x)=w41:i32)
    n25 = Negate(x=w33) -> (-x=w29:i16)
    n26 = property on="R2" class="DigNum (strict)"("Val(Sgnl)"=w29) -> ()  [unwired: 2 in, 2 out]
    n27 = property on="L2" class="DigNum (strict)"("Val(Sgnl)"=w30) -> ()  [unwired: 2 in, 2 out]
    n28 = feedback #1() -> (w73:bool)  [unwired: 1 in]
    n29 = feedback-in #1(w68) -> ()
    n30 = feedback #2() -> (w75:bool)  [unwired: 1 in]
    n31 = feedback-in #2(w67) -> ()
    n32 = Add(x=w40, y=w41) -> (x+y=w39:i32)
    n33 = feedback #3() -> (w61:bool)  [unwired: 1 in]
    n34 = feedback-in #3(w56) -> ()
    n35 = feedback #4() -> (w63:bool)  [unwired: 1 in]
    n36 = feedback-in #4(w55) -> ()
    n37 = Add(x=w43, y=w44) -> (x+y=w48:i32)
    n38 = Greater?(x=w68, y=w73) -> (0:w72:bool)
    n39 = Greater?(x=w67, y=w75) -> (0:w74:bool)
    n40 = Greater?(x=w56, y=w61) -> (0:w60:bool)
    n41 = Greater?(x=w55, y=w63) -> (0:w62:bool)
    n42 = call "Out of Range"("Operand 1"=w39) -> ("Result"=→"Left Joystick":dynamicdata)  [unwired: 9 in, 1 out]
    n43 = call "Out of Range"("Operand 1"=w48) -> ("Result"=→"Right Joystick":dynamicdata)  [unwired: 9 in, 1 out]
    n44 = call <vilib>:"Increment PtByPt.vi"("activate"=w72) -> ("counter"=w71:u32)  [unwired: 1 in, 1 out]
    n45 = call <vilib>:"Increment PtByPt.vi"("activate"=w74) -> ("counter"=w66:u32)  [unwired: 1 in, 1 out]
    n46 = call <vilib>:"Increment PtByPt.vi"("activate"=w60) -> ("counter"=w59:u32)  [unwired: 1 in, 1 out]
    n47 = call <vilib>:"Increment PtByPt.vi"("activate"=w62) -> ("counter"=w53:u32)  [unwired: 1 in, 1 out]
    n48 = To Double Precision Float(number=w71) -> (double precision float=w70:dbl)
    n49 = To Double Precision Float(number=w59) -> (double precision float=w58:dbl)
    n50 = Negate(x=w70) -> (-x=w69:dbl)
    n51 = Negate(x=w58) -> (-x=w54:dbl)
    n52 = Add(x=w69, y=w66) -> (x+y=w65:dbl)
    n53 = Add(x=w54, y=w53) -> (x+y=w57:dbl)
    n54 = Multiply(x=w65, y=w64) -> (x*y=w32:dbl)
    n55 = Multiply(x=w57, y=w52) -> (x*y=w31:dbl)
    n56 = property on="Power Limiter" class="Slide (strict)"("Val(Sgnl)"=w32) -> ()  [unwired: 2 in, 2 out]
    n57 = property on="VSP Speed" class="Slide (strict)"("Val(Sgnl)"=w31) -> ()  [unwired: 2 in, 2 out]
    n58 = property on="SIT_stopVI" class="Bool (strict)"() -> ("Value"=w36:bool)  [unwired: 2 in, 2 out]
    n59 = Wait (ms)(milliseconds to wait=u32 50) -> ()  [unwired: 1 out]
  }
  n60 = case shown="No Error" w26 {
    selector: w26 -> [_ w213]
    tunnel: w25 -> [w96 _]
    tunnel: w24 -> [w94 w212]
    tunnel: [w90 w213] -> w21
    tunnel: w17 -> [w93 _]
    tunnel: w16 -> [_ _]
    tunnel: [FALSE _] -> w15
    tunnel: w14 -> [w88 _]
    tunnel: w13 -> [w87 _]
    frame No Error {
      n61 = while {
        tunnel: w96 -> [w108]
        tunnel: [w106] -> w89
        shift-right: [w100] -> _
        shift-left: w93 -> [w104]
        shift-right: [w107] -> w95
        shift-left: w94 -> [w105]
        shift-right: [w97] -> _
        shift-left: w88 -> [w98]
        stop <- w99 stop-if-true
        n62 = event shown="[9] Timeout" {
          selector: w108 -> [_ _ _ _ _ _ _ _ _ _]
          dyn-events: _ -> [_ _ _ _ _ _ _ _ _ _]
          timeout: 100 -> [_ _ _ _ _ _ _ _ _ _]
          tunnel: ["SIT_stopVI" _ _ w143 _ _ _ _ _ _] -> w101
          tunnel: [_ w118 w130 w142 w155 w159 _ w170 _ w177] -> w102
          tunnel: w105 -> [w111 w116 w131 w144 w154 w158 w162 w169 _ w179]
          tunnel: w104 -> [w109 w117 w132 w145 w153 w156 w163 w165 w172 w178]
          tunnel: [w111 w116 w131 w144 w154 w158 w162 w169 w173 w179] -> w107
          tunnel: [w109 w117 w132 w145 w153 w156 w161 w165 w172 w178] -> w100
          tunnel: [w110 SIT_Sim_State."Running" ("State") SIT_Sim_State."Paused" ("State") SIT_Sim_State."Stopped" ("State") w152 w157 w160 w164 w171 w175] -> w97
          tunnel: w98 -> [w110 _ _ _ w152 w157 w160 w164 w171 w176]
          event "SIT_stopVI": Value Change {
            n63 = event-data() -> ()  [unwired: 2 out]
          }
          event "SIT_Run": Value Change {
            n64 = event-data() -> ("OldVal"=w114:bool, "NewVal"=w115:bool)  [unwired: 1 out]
            n65 = local read "SIT_Pause"() -> (w121:bool)
            n66 = Equal?(x=w114, y=w115) -> (x = y?=w119:bool)
            n67 = Not(x=w121) -> (.not. x?=w122:bool)
            n68 = And(x=w122, y=w119) -> (x .and. y?=w120:bool)
            n69 = case shown="False" w120 {
              tunnel: [w126 _] -> w118
              tunnel: w117 -> [w125 _]
              tunnel: w116 -> [w124 _]
              frame False {
                n70 = call <vilib>:"sit Run Model.vi"("SIT Meta Info"=w124, "SIT Client Op Refs"=w125) -> ("error out"=w126:errorcluster, "Status"=w123:string)  [unwired: 6 in, 2 out]
                n71 = local write "SIT_Status"(w123) -> ()
              }
              frame True {
                # "Ignore value change if it is\nto the same value"
              }
            }
          }
          event "SIT_Pause": Value Change {
            n72 = event-data() -> ("OldVal"=w128:bool, "NewVal"=w129:bool)  [unwired: 1 out]
            n73 = Equal?(x=w128, y=w129) -> (x = y?=w133:bool)
            n74 = case shown="False" w133 {
              tunnel: [w138 _] -> w130
              tunnel: w132 -> [w137 _]
              tunnel: w131 -> [w136 _]
              tunnel: w129 -> [w135 _]
              frame False {
                n75 = call <vilib>:"sit Pause Model.vi"("Pause Button Value"=w135, "SIT Meta Info"=w136, "SIT Client Op Refs"=w137) -> ("error out"=w138:errorcluster, "Status"=w134:string)  [unwired: 3 in, 4 out]
                n76 = local write "SIT_Status"(w134) -> ()
              }
              frame True {
                # "Ignore value change if it is\nto the same value"
              }
            }
          }
          event "SIT_Stop": Value Change {
            n77 = event-data() -> ("OldVal"=w140:bool, "NewVal"=w141:bool)  [unwired: 1 out]
            n78 = Equal?(x=w140, y=w141) -> (x = y?=w146:bool)
            n79 = case shown="False" w146 {
              tunnel: [w151 _] -> w142
              tunnel: [w148 _] -> w143
              tunnel: w144 -> [w150 _]
              tunnel: w145 -> [w149 _]
              frame False {
                n80 = call <vilib>:"sit Stop Model.vi"("SIT Meta Info"=w150, "SIT Client Op Refs"=w149) -> ("error out"=w151:errorcluster, "Status"=w147:string, "Stop VI?"=w148:bool)  [unwired: 4 in, 3 out]
                n81 = local write "SIT_stopVI"(w148) -> ()
                n82 = local write "SIT_Status"(w147) -> ()
              }
              frame True {
                # "Ignore value change if it is\nto the same value"
              }
            }
          }
          event "SIT_Details": Value Change {
            n83 = event-data() -> ()  [unwired: 2 out]
            n84 = call <vilib>:"sit Launch Details Dialog.vi"("SIT Meta Info in"=w154, "SIT Client Op Refs"=w153) -> ("error out"=w155:errorcluster)  [unwired: 1 in, 8 out]
          }
          event "SIT_Remap": Value Change {
            n85 = event-data() -> ()  [unwired: 2 out]
            n86 = call <vilib>:"sit Launch Remap Dialog.vi"("SIT Meta Info in"=w158, "SIT Client Op Refs"=w156) -> ("error out"=w159:errorcluster)  [unwired: 2 in, 7 out]
          }
          event "SIT_RVE": Value Change {
            n87 = event-data() -> ()  [unwired: 2 out]
            n88 = call <vilib>:"RVE.vi"("SIT_Meta_Info"=w162, "SIT Client Op Refs in"=w163) -> ("SIT Client Op Refs out"=w161:T11)  [unwired: 9 out]
          }
          event Value Change {
            n89 = event-data() -> ("NewVal"=w166:variant, "OldVal"=w167:variant, "CtlRef"=w168:refnum<vi>)  [unwired: 1 out]
            n90 = call <vilib>:"sit Send New Control Value.vi"("Control New Value"=w166, "Control Old Value"=w167, "Control Ref"=w168, "SIT Client Op Refs"=w165, "SIT_Meta_Info"=w169) -> ("error out"=w170:errorcluster)  [unwired: 4 in, 2 out]
          }
          event Value Change {
            n91 = event-data() -> ("NewVal"=w173:T2)  [unwired: 1 out]
          }
          event Timeout {
            n92 = event-data() -> ()  [unwired: 2 out]
            n93 = call <vilib>:"sit Check State Change.vi"("Old State in"=w176, "SIT Client Op Refs"=w178) -> ("error out"=w177:errorcluster, "Status String"=w174:string, "New State out"=w175:T13)  [unwired: 7 out]
            n94 = local write "SIT_Status"(w174) -> ()
          }
        }
        n95 = call <vilib>:"sit Check to Stop Client.vi"("error in (no error)"=w102, "User Stop?"=w101) -> ("error out"=w106:errorcluster, "Stop?"=w99:bool)  [unwired: 1 in, 7 out]
      }
      n96 = while "Read Loop" {
        tunnel: [w190] -> w91
        tunnel: w87 -> [w180]
        i -> [w187]
        stop <- w188 stop-if-true
        n97 = call <vilib>:"sit Signal Probe Data.vi"("TCP Conn and Queue"=w180) -> ("error out"=w183:errorcluster, "Dimensions"=w184:i32[], "Raw Data"=w185:dbl[][], "dup TCP Conn and Queue"=w186:T10, "Valid Data?"=w181:bool, "Options out"=w182:u32)  [unwired: 4 in, 1 out]
        n98 = case shown="True" w181 {
          tunnel: w185 -> [_ w201]
          tunnel: w184 -> [_ w200]
          tunnel: w186 -> [w193 w199]
          tunnel: w183 -> [w196 w198]
          tunnel: [w195 w198] -> w189
          tunnel: w182 -> [w197 _]
          tunnel: w187 -> [w194 _]
          frame False {
            # "Probe did not return valid data, do not update indicators"
            n99 = local read "SIT_Meta_Info"() -> (w192:T2)
            n100 = call <vilib>:"sit Check For Data Loss Error.vi"("Iteration"=w194, "SIT Meta Info"=w192, "error in (no error)"=w196, "Options"=w197, "TCP Conn and Queue"=w193) -> ("error out"=w195:errorcluster)  [unwired: 6 out]
          }
          frame True {
            n101 = for {
              tunnel: w201 -> [w211]
              tunnel: "SIT_Indicator_Indices" -> [w207] mode=indexing
              tunnel: w200 -> [w210]
              tunnel: w199 -> [w208]
              i -> [w209]
              n102 = call <vilib>:"sit Get Current Data.vi"("Indicator Index Cluster"=w207, "Iteration"=w209, "Dimensions"=w210, "Raw Data"=w211, "Conn and Queue"=w208) -> ("Timestamps"=w204:dbl[], "Last Row"=w205:i32, "Current Data"=w206:dbl[][], "Indicator Index"=w203:i32)  [unwired: 1 in, 2 out]
              n103 = case "SIT_Indicator_Cases" shown="-1, Default" w203 {
                tunnel: w206 -> [_]
                tunnel: w205 -> [_]
                tunnel: w204 -> [_]
                frame -1, Default {
                }
              }
            }
          }
        }
        n104 = call <vilib>:"sit Check to Stop Client.vi"("error in (no error)"=w189) -> ("error out"=w190:errorcluster, "Stop?"=w188:bool)  [unwired: 2 in, 7 out]
        n105 = Wait (ms)(milliseconds to wait=u32 50) -> ()  [unwired: 1 out]
      }
      n106 = local write "SIT_Meta_Info"(w95) -> ()
      n107 = call <vilib>:"sit Merge SIT Client Errors.vi"("Bottom Loop Error"=w91, "Top Loop Error"=w89) -> ("Resulting Error"=w90:errorcluster)  [unwired: 9 out]
    }
    frame Error {
      # "User canceled target selection (or an error occurred on Init)...don't run the client"
      n108 = local write "SIT_Meta_Info"(w212) -> ()
    }
  }
  n109 = local write "SIT_stopVI"(w15) -> ()
  n110 = call <vilib>:"sit Clear Client.vi"("error in (no error)"=w21, "SIT Client Op Refs"=w17) -> ("error out"=w18:errorcluster)  [unwired: 9 out]
  n111 = call <vilib>:"sit Check to Stop Client.vi"("Reset Stop?"=TRUE ("Clear Item?"), "error in (no error)"=w18) -> ("error out"=w10:errorcluster)  [unwired: 1 in, 8 out]
  n112 = call <vilib>:"sit Check Run-Time System.vi"("error in"=w10) -> ("Run Time System?"=w9:bool)  [unwired: 10 out]
  n113 = Quit LabVIEW(quit? (T)=w9) -> ()
  n114 = call-poly <vilib>:"Close Input Device.vi"("error in (no error)"=w2, "device ID"=w3) -> ("error out"=w1:errorcluster)  [unwired: 8 in]
  n115 = call <vilib>:"General Error Handler.vi"("error in (no error)"=w1) -> ()  [unwired: 10 in, 5 out]
